vi "Global Variables.vi"() -> ()   [LabVIEW 2014]
doc: "This global VI can contain as many global variables as you need. Place a control on the panel, give it a good name. To read or write to it from a VI, drag the icon to the diagram of that VI. You can also drag from the project. Click on the node to change which global you access. You shouldn't have multiple locations writing to a global or it will cause a race-condition."
uses:
  <vilib>/Rock Robotics/WPI/DriverStation/WPI_DriverStationRobotMode2.ctl
panel:
  in  "Lidar Active":bool
  out "Lift DPad Control":i16
  out "Lift Joystick Control":dbl=3.0
  in  "Lift Encoder Reset":bool
  in  "Lift Sequence Done":bool
  in  "Roller Arms In":bool
  in  "Rollers Out":bool
  in  "Rollers In":bool
  out "Driver Back":bool
  out "Lift Offset":dbl=3.0
  out "Lift Speed":dbl=0.5
  in  "Lift Stop":bool
  out "Lift Height":dbl
  in  "Lift PID Done":bool
  out "Lift Inches":dbl
  out "Lift Inches Target":dbl
  in  "Step":bool
  in  "Pickup Floor":bool
  in  "Pickup":bool
  in  "Place":bool
  in  "Tote 3":bool
  in  "Tote 2":bool
  in  "Tote 1":bool
  in  "Lift E-Stop":bool
  out "Drive Enc BR":dbl
  out "Drive Enc BL":dbl
  out "Drive Enc FR":dbl
  out "Drive Enc FL":dbl
  out "Driver Start":bool
  out "Heading to Maintain":dbl
  out "NavX Yaw":dbl
  out "Driver Joystick X2":dbl
  out "Driver Joystick Y1":dbl
  out "Driver Joystick X1":dbl
  out "Rot BR":dbl
  out "Drive BR":dbl
  out "Rot BL":dbl
  out "Drive BL":dbl
  out "Rot FR":dbl
  out "Drive FR":dbl
  out "Rot FL":dbl
  out "Drive FL":dbl
  in  "Robot Mode":T1=enum."Teleop Disabled"
  # "Sensors"
  # "Lift"
  # "Misc"
  # "Drive Motors"
  # "Driver Controller"
  # "Intake & Eject"
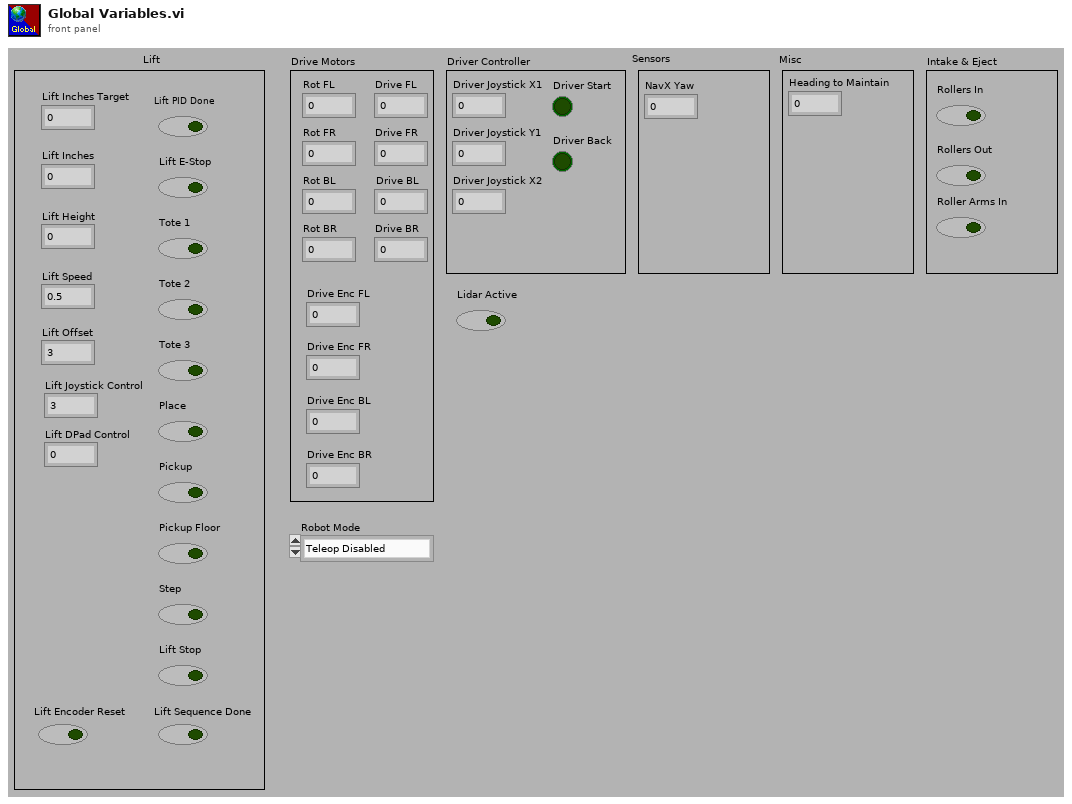
[diagram p1: front panel]
types:
  T1 = typedef "WPI_DriverStationRobotMode2.ctl" = enum16{"Autonomous Disabled", "Autonomous Enabled", "Teleop Disabled", "Teleop Enabled", "Disconnected", "Finish", "Test Disabled", "Test Enabled", "Emergency Stopped"}
diagram:
